vi "Destroy.vi"(0 "reference in":refnum<class "File Controller.lvclass">, 5 "error in (no error)":errorcluster) -> (14 "reference out":refnum<class "File Controller.lvclass">, 19 "error out":errorcluster)   [LabVIEW 2015, in "File Controller.lvclass"]
doc: "Destructor."
uses:
  File Controller.lvclass
  <vilib>/addons/_AddQ/G#Object/G#Object.lvclass
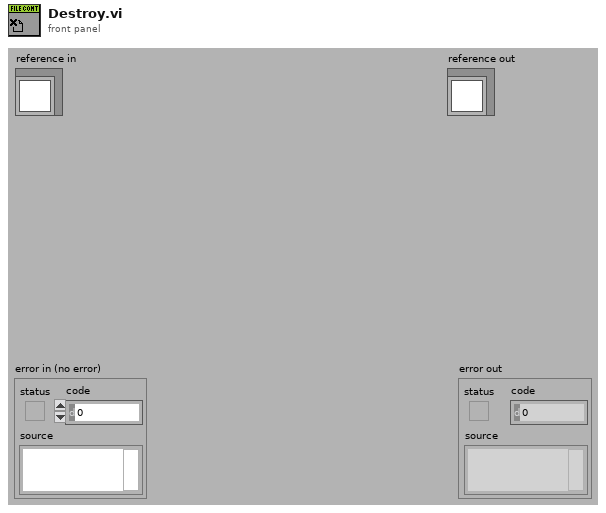
[diagram p1: front panel]
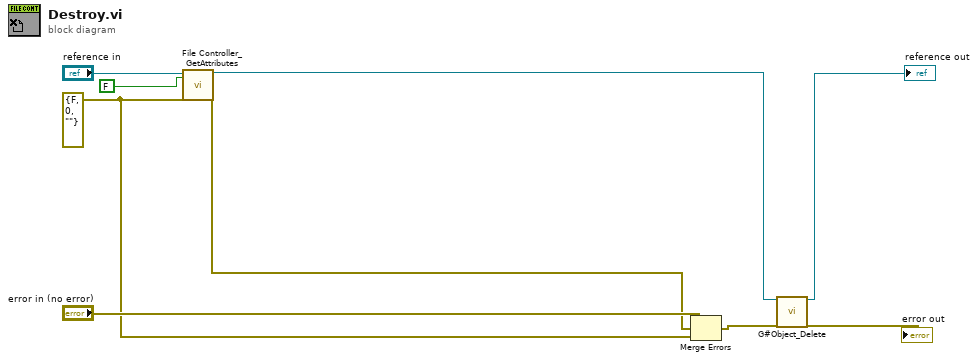
[diagram p0: block diagram]
diagram:
  w7 = errorcluster {"status"=FALSE, "code"=0, "source"=""} ("error in (no error)")
  n1 = call "File Controller_GetAttributes.vi"("reference in"="reference in", "return data? (T)"=FALSE ("simple info"), "error in (no error)"=w7) -> ("reference out"=w4:refnum<class "File Controller.lvclass">, "error out"=w1:errorcluster)  [unwired: 13 in, 2 out]
  n2 = Merge Errors("error in (no error)", w1, w7) -> (w6:errorcluster)
  n3 = call <vilib>:"G#Object_Delete.vi"("reference in"=w4, "error in (no error)"=w6) -> ("reference out"=→"reference out":refnum<class "File Controller.lvclass">, "error out"=→"error out":errorcluster)  [unwired: 16 in]
